vi "Naplófájl.vi"(6 "Index":i32, 9 "Dátum(string)":string, 10 "Összekevert tömb":string[](array[string]), 11 "Eredeti tömb":string[][](array[string])) -> (3 "Kész naplófájl(2D Tömb)":string[][](array[string]))   [LabVIEW 2014]
doc: "Az eredeti fájl átalakítja úgy, hogy az 1. oszlop fejlécének helyére beírja a dátumot és az idõt, a 2. oszlop fejlécét üresen hadja, és az ezutáni sorokba beírja a párokat."
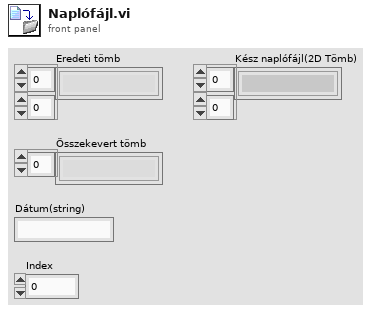
[diagram p1: front panel]
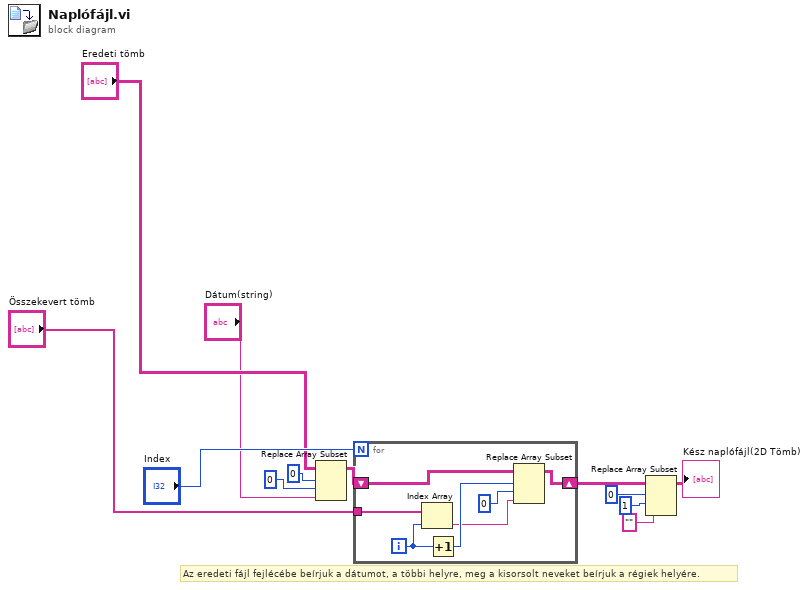
[diagram p0: block diagram]
diagram:
  # "Az eredeti fájl fejlécébe beírjuk a dátumot, a többi helyre, meg a kisorsolt neveket beírjuk a régiek helyére."
  n1 = Replace Array Subset(array="Eredeti tömb", new element="Dátum(string)", index (row)=0, index (col)=0 ("disabled index (col)")) -> (w6:string[][])
  n2 = for {
    N: "Index" -> [_]
    shift-right: [w15] -> w10
    shift-left: w6 -> [w16]
    tunnel: "Összekevert tömb" -> [w14]
    i -> [w19]
    n3 = Index Array(array=w14, index=w19) -> (element=w13:string)
    n4 = Increment(x=w19) -> (x+1=w17:i32)
    n5 = Replace Array Subset(array=w16, new element=w13, index (row)=w17, index (col)=0 ("disabled index (col)")) -> (w15:string[][])
  }
  n6 = Replace Array Subset(array=w10, new element="" ("new element/subarray"), index (row)=0 ("disabled index (row)"), index (col)=1 ("disabled index (col)")) -> (→"Kész naplófájl(2D Tömb)":string[][])
